vi "2DRasterScanWithScopeComm.vi"() -> ()   [LabVIEW 2015]
panel:
  out "error out 3":errorcluster
  out "error out 2":errorcluster
  in  "Z safe rretract":sgl
  in  "MG17Motor Z axis":refnum<k7>(container)
  in  "Home Z?":bool caption="Do this each time LabVIEW\n is opened, controllers are\n unplugged, or stages are\n         disconnected"
  in  "Z-Axis Serial":i32=27501169
  in  "Safe retract?":bool=TRUE
  in  "X safe rretract":sgl
  in  "Y safe retract":sgl
  out "Y error":errorcluster
  in  "Base filename":string="README" caption="Filename"
  in  "Save Each Point":bool=TRUE
  in  "X-Axis Serial":i32=45869591
  in  "Y-Axis Serial":i32=27501169
  out "Number of movements for Y stage":sgl=21.0
  in  "Distance from center X axis (mm)":dbl=15.0 step=0.001
  in  "Movement Step Size X axis (mm)":sgl=1.0 step=0.001
  in  "Channel Select":T1(ring)=enum."Channel 3"
  in  "Selected Directory":path=path "C:/Users/admin.WIN10DC20170225/Documents/Hydrophone Data/Test"
  in  "Stage Max Velocity (mm/s)":sgl=1.5
  in  "Stage Acceleration (mm/s²)":sgl=1.0
  in  "Stage Minimum Velocity (mm/s)":sgl
  in  "Center point Y axis (mm)":dbl=25.0 step=0.001 format="%#_13g"
  in  "Center point X axis (mm)":dbl=80.0 step=0.001 format="%#_13g"
  out "Number of movements for X stage":sgl=31.0
  in  "Distance from center Y axis (mm)":dbl=10.0 step=0.001
  in  "MG17Motor X axis":refnum<k7>(container)
  in  "Home stages\nbefore scanning":bool caption="Do this each time LabVIEW\n is opened, controllers are\n unplugged, or stages are\n         disconnected"
  in  "error in (no error)":errorcluster
  in  "MG17Motor Y axis":refnum<k7>(container)
  out "Current position in line":i32=1
  out "Current line number":i32=1
  in  "Movement Step Size Y axis (mm)":sgl=1.0 step=0.001
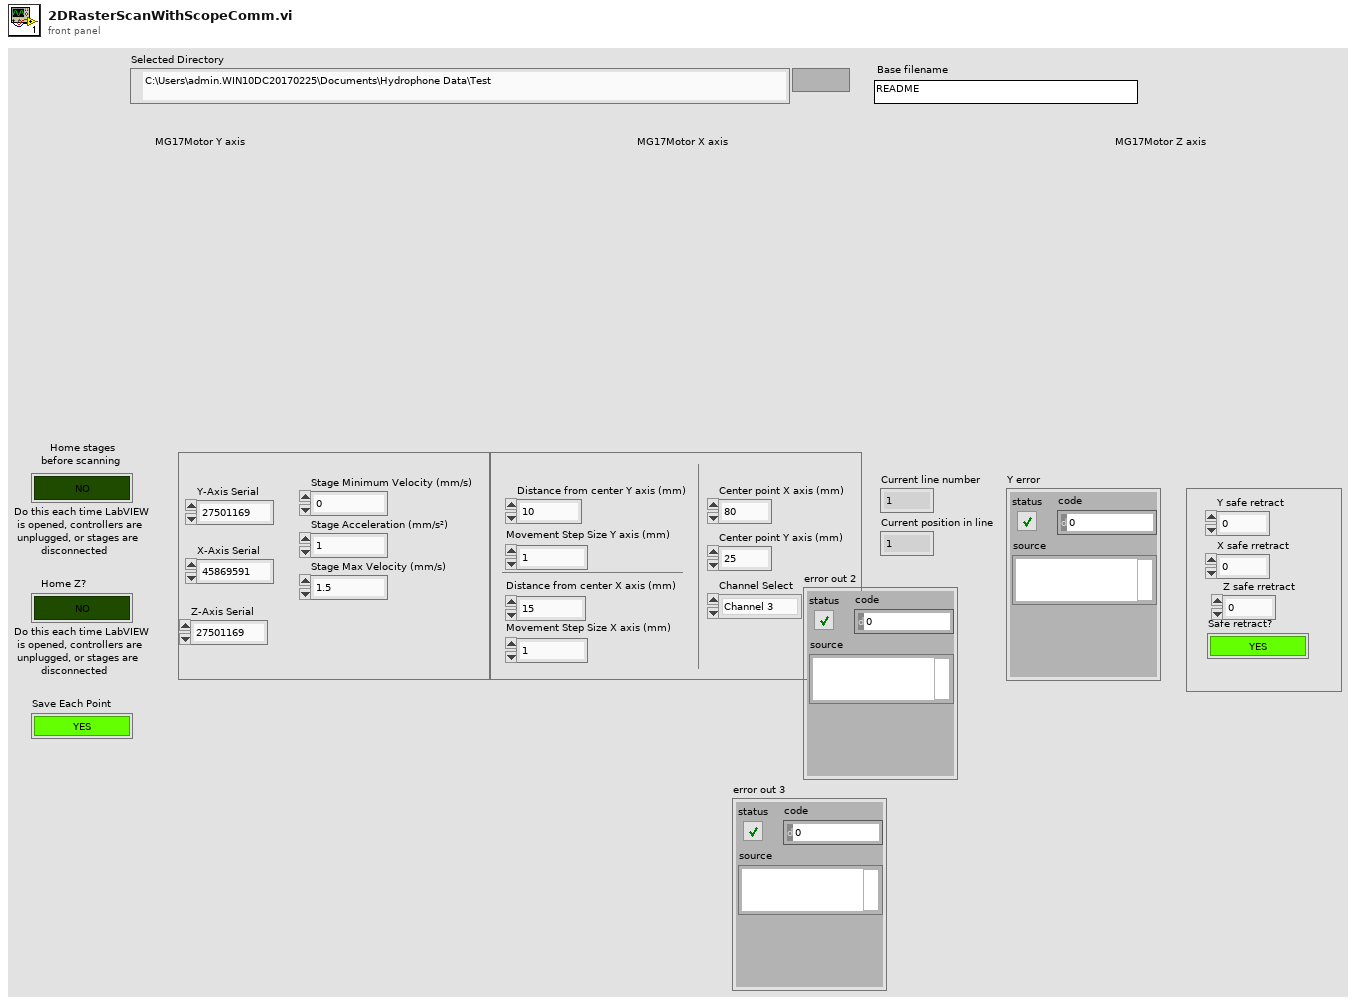
[diagram p1: front panel]
types:
  T1 = enum16{"Trace D", "Trace C", "Trace B", "Trace A", "Channel 4", "Channel 3", "Channel 2", "Channel 1"}
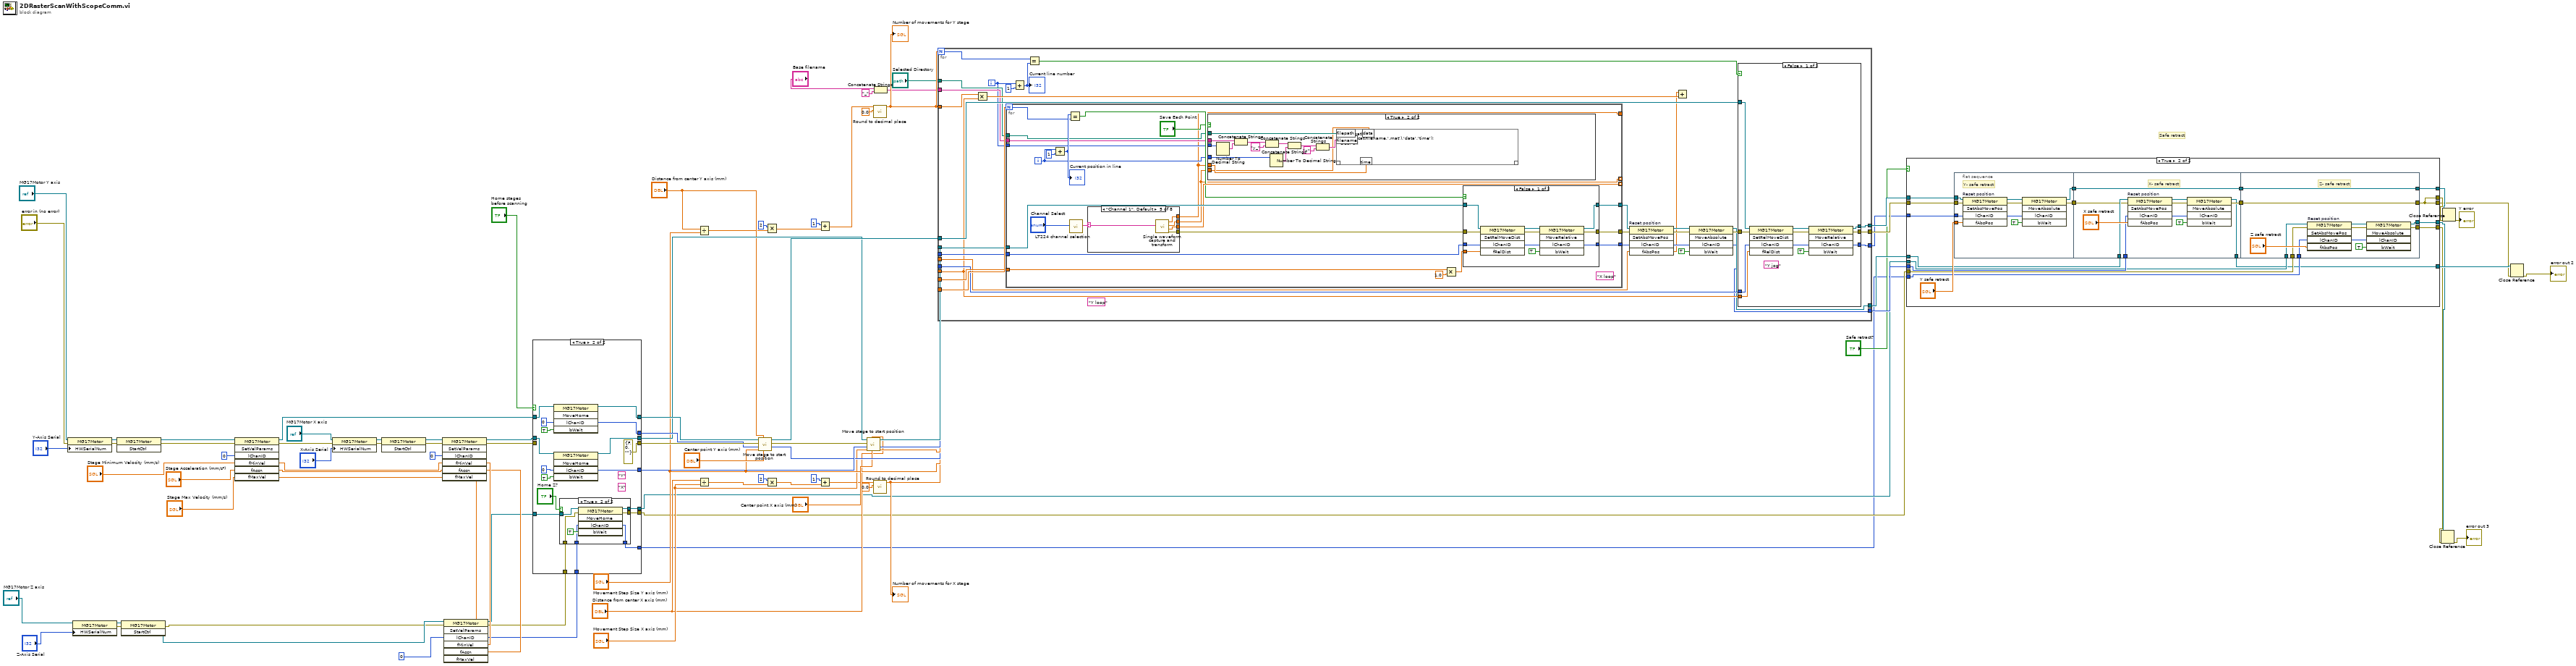
[diagram p0: block diagram]
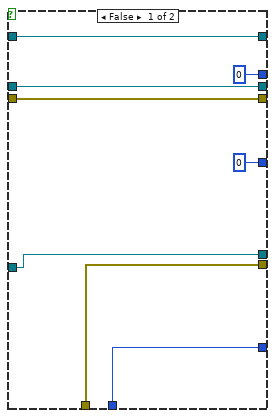
[diagram p3: hidden frame]
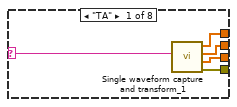
[diagram p8: hidden frame]
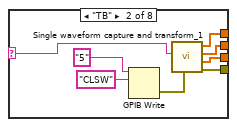
[diagram p9: hidden frame]
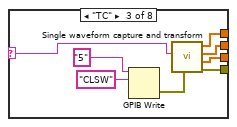
[diagram p10: hidden frame]
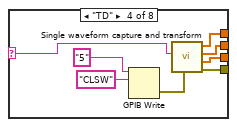
[diagram p11: hidden frame]
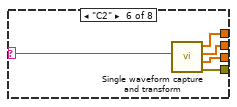
[diagram p12: hidden frame]
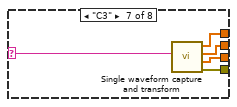
[diagram p13: hidden frame]
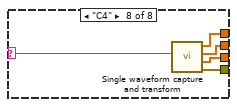
[diagram p14: hidden frame]
diagram:
  # "Safe retract"
  n1 = property on="Property Node" class="MG17Motor"(reference="MG17Motor Y axis", error in="error in (no error)", "HWSerialNum"="Y-Axis Serial") -> (reference out=w91:refnum<k7>, error out=w90:errorcluster)
  n2 = property on="Property Node" class="MG17Motor"(reference="MG17Motor Z axis", "HWSerialNum"="Z-Axis Serial") -> (reference out=w20:refnum<k7>, error out=w21:errorcluster)  [unwired: 1 in]
  n3 = invoke class="MG17Motor" method="StartCtrl"(reference=w91, error in=w90) -> (reference out=w83:refnum<k7>, error out=w84:errorcluster)  [unwired: 1 in, 1 out]
  n4 = invoke class="MG17Motor" method="StartCtrl"(reference=w20, error in=w21) -> (reference out=w15:refnum<k7>, error out=w14:errorcluster)  [unwired: 1 in, 1 out]
  n5 = invoke class="MG17Motor" method="SetVelParams"(reference=w83, error in=w84, "lChanID"=0, "fMinVel"="Stage Minimum Velocity (mm/s)", "fAccn"="Stage Acceleration (mm/s²)", "fMaxVel"="Stage Max Velocity (mm/s)") -> (reference out=w72:refnum<k7>, error out=w73:errorcluster, "fMinVel"=w53:sgl, "fAccn"=w52:sgl, "fMaxVel"=w51:sgl)  [unwired: 1 in, 2 out]
  n6 = property on="Property Node" class="MG17Motor"(reference="MG17Motor X axis", error in=w73, "HWSerialNum"="X-Axis Serial") -> (reference out=w86:refnum<k7>, error out=w85:errorcluster)
  n7 = invoke class="MG17Motor" method="StartCtrl"(reference=w86, error in=w85) -> (reference out=w82:refnum<k7>, error out=w75:errorcluster)  [unwired: 1 in, 1 out]
  n8 = invoke class="MG17Motor" method="SetVelParams"(reference=w82, error in=w75, "lChanID"=0, "fMinVel"=w53, "fAccn"=w52, "fMaxVel"=w51) -> (reference out=w81:refnum<k7>, error out=w74:errorcluster, "fMinVel"=w19:sgl, "fAccn"=w18:sgl, "fMaxVel"=w17:sgl)  [unwired: 1 in, 2 out]
  n9 = invoke class="MG17Motor" method="SetVelParams"(reference=w15, error in=w14, "lChanID"=0, "fMinVel"=w19, "fAccn"=w18, "fMaxVel"=w17) -> (reference out=w12:refnum<k7>, error out=w11:errorcluster, "lChanID"=w5:i32)  [unwired: 1 in, 4 out]
  n10 = case shown="True" "Home stages\nbefore scanning" {
    tunnel: [w97 w114] -> w62
    tunnel: [w98 w113] -> w68
    tunnel: [0 ("lChanID") w112] -> w63
    tunnel: [0 ("lChanID") w111] -> w66
    tunnel: [w96 errorcluster {"status"=FALSE, "code"=0, "source"=""} ("error out")] -> w67
    tunnel: w72 -> [w98 w109]
    tunnel: w81 -> [w97 w108]
    tunnel: w74 -> [w96 _]
    tunnel: w12 -> [w95 w106]
    tunnel: w11 -> [w94 w105]
    tunnel: [w95 w104] -> w9
    tunnel: [w94 w103] -> w8
    tunnel: w5 -> [w93 w102]
    tunnel: [w93 w101] -> w4
    frame False {
    }
    frame True {
      (unwired) "X"
      (unwired) "Y"
      n11 = invoke class="MG17Motor" method="MoveHome"(reference=w109, "lChanID"=0, "bWait"=TRUE) -> (reference out=w113:refnum<k7>, "lChanID"=w111:i32)  [unwired: 2 in, 3 out]
      n12 = invoke class="MG17Motor" method="MoveHome"(reference=w108, "lChanID"=0, "bWait"=TRUE) -> (reference out=w114:refnum<k7>, "lChanID"=w112:i32)  [unwired: 2 in, 3 out]
      n13 = case shown="True" "Home Z?" {
        tunnel: w106 -> [w121 w127]
        tunnel: w105 -> [w120 w126]
        tunnel: [w121 w125] -> w104
        tunnel: [w120 w124] -> w103
        tunnel: w102 -> [w119 w123]
        tunnel: [w119 w122] -> w101
        frame False {
        }
        frame True {
          n14 = invoke class="MG17Motor" method="MoveHome"(reference=w127, error in=w126, "lChanID"=w123, "bWait"=TRUE) -> (reference out=w125:refnum<k7>, error out=w124:errorcluster, "lChanID"=w122:i32)  [unwired: 1 in, 2 out]
        }
      }
    }
  }
  n15 = Divide(x="Distance from center Y axis (mm)", y="Movement Step Size Y axis (mm)") -> (x/y=w56:dbl)
  n16 = Divide(x="Distance from center X axis (mm)", y="Movement Step Size X axis (mm)") -> (x/y=w47:dbl)
  n17 = call "Move stage to start position.vi"("Center point of axis (mm)"="Center point Y axis (mm)", "Distance from center (mm)"="Distance from center Y axis (mm)", "Movement Step Size (mm)"="Movement Step Size Y axis (mm)", "lChanID"=w66, "error in"=w67, "reference in"=w68) -> ("lChanID out"=w57:i32, "error out"=w64:errorcluster, "reference out"=w65:refnum<k7>)  [unwired: 2 in, 1 out]
  n18 = Multiply(x=2, y=w56) -> (x*y=w70:dbl)
  n19 = Multiply(x=2, y=w47) -> (x*y=w48:dbl)
  n20 = Add(x=1, y=w70) -> (x+y=w40:dbl)
  n21 = Add(x=1, y=w48) -> (x+y=w41:dbl)
  n22 = call "Move stage to start position.vi"("Center point of axis (mm)"="Center point X axis (mm)", "Distance from center (mm)"="Distance from center X axis (mm)", "Movement Step Size (mm)"="Movement Step Size X axis (mm)", "lChanID"=w63, "error in"=w64, "reference in"=w62) -> ("Start position out"=w58:sgl, "lChanID out"=w59:i32, "reference out"=w60:refnum<k7>)  [unwired: 2 in, 1 out]
  n23 = call "Round to decimal place.vi"("Power of ten"=0.0, "Number to round"=w40) -> ("Rounded number"=w42:dbl)  [unwired: 8 in, 1 out]
  "Number of movements for Y stage" <- w42
  n24 = call "Round to decimal place.vi"("Power of ten"=0.0, "Number to round"=w41) -> ("Rounded number"=w43:dbl)  [unwired: 8 in, 1 out]
  "Number of movements for X stage" <- w43
  n25 = Concatenate Strings("Base filename", "_" ("string")) -> (w33:string)
  n26 = for {
    N: w42 -> [w149]
    tunnel: "Movement Step Size Y axis (mm)" -> [w154]
    tunnel: w43 -> [w159]
    tunnel: [w147] -> w30
    tunnel: [w146] -> w3
    tunnel: "Movement Step Size Y axis (mm)" -> [w139]
    tunnel: w65 -> [w145]
    tunnel: w60 -> [w144]
    tunnel: w59 -> [w143]
    tunnel: w58 -> [w142]
    tunnel: w57 -> [w141]
    tunnel: w42 -> [w138]
    tunnel: w33 -> [w134]
    tunnel: "Selected Directory" -> [w133]
    tunnel: [w131] -> w28
    tunnel: [w130] -> w29
    tunnel: [w129] -> w27
    i -> [w132]
    (unwired) "Y loop"
    n27 = Multiply(x=w138, y=w139) -> (x*y=w140:dbl)
    n28 = for {
      N: w159 -> [w181]
      tunnel: w154 -> [w188]
      tunnel: [w174] -> _
      tunnel: [w192] -> w135
      tunnel: [w193] -> w152
      tunnel: [w191] -> w151
      tunnel: [w185] -> _ mode=indexing
      tunnel: w144 -> [w189]
      tunnel: w143 -> [w190]
      tunnel: [w179] -> _ mode=indexing
      tunnel: w134 -> [w180]
      tunnel: w133 -> [w178]
      tunnel: w132 -> [w176]
      i -> [w177]
      (unwired) "X loop"
      n29 = Add(x=w177, y=1) -> (x+y=w182:i32)
      "Current position in line" <- w182
      n30 = Equal?(x=w182, y=w181) -> (x = y?=w183:bool)
      n31 = call "LT224 channel selection.vi"("Channel Select"="Channel Select") -> ("Selected channel"=w186:string)  [unwired: 10 in]
      n32 = case shown="\"Channel 1\", Default" w186 {
        selector: w186 -> [w226 w231 w239 w247 w255 w260 w265 w270]
        tunnel: [w229 w237 w245 w253 w258 w263 w268 w273] -> w184
        tunnel: [w228 w236 w244 w252 w257 w262 w267 w272] -> w185
        tunnel: [w227 w235 w243 w251 w256 w261 w266 w271] -> w174
        tunnel: [w225 w230 w238 w246 w254 w259 w264 w269] -> w179
        frame "TA" {
          n33 = call "Single waveform capture and transform_1.vi"("channel name (\"\")"=w226) -> ("error out"=w229:errorcluster, "Transformed waveform vector"=w228:dbl[], "waveform vector"=w225:dbl[], "Time vector"=w227:dbl[])  [unwired: 7 in]
        }
        frame "TB" {
          n34 = GPIB Write(0:"5" ("address string"), 1:"CLSW" ("data")) -> (6:w233:errorcluster)  [unwired: 3 in, 1 out]
          n35 = call "Single waveform capture and transform_1.vi"("error in"=w233, "channel name (\"\")"=w231) -> ("error out"=w237:errorcluster, "Transformed waveform vector"=w236:dbl[], "waveform vector"=w230:dbl[], "Time vector"=w235:dbl[])  [unwired: 6 in]
        }
        frame "TC" {
          n36 = GPIB Write(0:"5" ("address string"), 1:"CLSW" ("data")) -> (6:w241:errorcluster)  [unwired: 3 in, 1 out]
          n37 = call "Single waveform capture and transform.vi"("error in"=w241, "channel name (\"\")"=w239) -> ("error out"=w245:errorcluster, "Transformed waveform vector"=w244:dbl[], "waveform vector"=w238:dbl[], "Time vector"=w243:dbl[])  [unwired: 6 in]
        }
        frame "TD" {
          n38 = GPIB Write(0:"5" ("address string"), 1:"CLSW" ("data")) -> (6:w249:errorcluster)  [unwired: 3 in, 1 out]
          n39 = call "Single waveform capture and transform.vi"("error in"=w249, "channel name (\"\")"=w247) -> ("error out"=w253:errorcluster, "Transformed waveform vector"=w252:dbl[], "waveform vector"=w246:dbl[], "Time vector"=w251:dbl[])  [unwired: 6 in]
        }
        frame "Channel 1", Default {
          n40 = call "Single waveform capture and transform.vi"("channel name (\"\")"=w255) -> ("error out"=w258:errorcluster, "Transformed waveform vector"=w257:dbl[], "waveform vector"=w254:dbl[], "Time vector"=w256:dbl[])  [unwired: 7 in]
        }
        frame "C2" {
          n41 = call "Single waveform capture and transform.vi"("channel name (\"\")"=w260) -> ("error out"=w263:errorcluster, "Transformed waveform vector"=w262:dbl[], "waveform vector"=w259:dbl[], "Time vector"=w261:dbl[])  [unwired: 7 in]
        }
        frame "C3" {
          n42 = call "Single waveform capture and transform.vi"("channel name (\"\")"=w265) -> ("error out"=w268:errorcluster, "Transformed waveform vector"=w267:dbl[], "waveform vector"=w264:dbl[], "Time vector"=w266:dbl[])  [unwired: 7 in]
        }
        frame "C4" {
          n43 = call "Single waveform capture and transform.vi"("channel name (\"\")"=w270) -> ("error out"=w273:errorcluster, "Transformed waveform vector"=w272:dbl[], "waveform vector"=w269:dbl[], "Time vector"=w271:dbl[])  [unwired: 7 in]
        }
      }
      n44 = case shown="True" "Save Each Point" {
        tunnel: w180 -> [_ w202]
        tunnel: w179 -> [_ w197]
        tunnel: w178 -> [_ w200]
        tunnel: w177 -> [_ w210]
        tunnel: w176 -> [_ w204]
        tunnel: w174 -> [_ w198]
        frame False {
        }
        frame True {
          n45 = Number To Decimal String(number=w204) -> (decimal integer string=w201:string)  [unwired: 1 in]
          n46 = Concatenate Strings(w202, w201) -> (w209:string)
          n47 = Concatenate Strings(w209, "y_" ("string")) -> (w207:string)
          n48 = Number To Decimal String(number=w210) -> (decimal integer string=w203:string)  [unwired: 1 in]
          n49 = Concatenate Strings(w207, w203) -> (w205:string)
          n50 = Concatenate Strings(w205, "x" ("string")) -> (w199:string)
          n51 = script code="cd(filepath)\nsave(strcat(filename,'.mat'),'data','time');\nclear all"("filename"=w199, "filepath"=w200, "time"=w198, "data"=w197) -> ()  [unwired: 1 in, 1 out]
        }
      }
      n52 = Multiply(x=w188, y=sgl 1.0) -> (x*y=w195:sgl)
      n53 = case shown="False" w183 {
        tunnel: w195 -> [w221 _]
        tunnel: [w216 w222] -> w193
        tunnel: [w215 w224] -> w192
        tunnel: [w214 w223] -> w191
        tunnel: w190 -> [w213 w223]
        tunnel: w189 -> [w212 w222]
        tunnel: w184 -> [w211 w224]
        frame False {
          n54 = invoke class="MG17Motor" method="SetRelMoveDist"(reference=w212, error in=w211, "lChanID"=w213, "fRelDist"=w221) -> (reference out=w219:refnum<k7>, error out=w218:errorcluster, "lChanID"=w220:i32)  [unwired: 1 in, 2 out]
          n55 = invoke class="MG17Motor" method="MoveRelative"(reference=w219, error in=w218, "lChanID"=w220, "bWait"=TRUE) -> (reference out=w216:refnum<k7>, error out=w215:errorcluster, "lChanID"=w214:i32)  [unwired: 1 in, 2 out]
        }
        frame True {
        }
      }
    }
    n56 = Add(x=w132, y=1) -> (x+y=w136:i32)
    "Current line number" <- w136
    n57 = Equal?(x=w149, y=w136) -> (x = y?=w150:bool)
    n58 = invoke on="Reset position" class="MG17Motor" method="SetAbsMovePos"(reference=w152, error in=w135, "lChanID"=w151, "fAbsPos"=w142) -> (reference out=w155:refnum<k7>, error out=w157:errorcluster, "lChanID"=w156:i32, "fAbsPos"=w137:sgl)  [unwired: 1 in, 1 out]
    n59 = Add(x=w137, y=w140) -> ()  [unwired: 1 out]
    n60 = invoke class="MG17Motor" method="MoveAbsolute"(reference=w155, error in=w157, "lChanID"=w156, "bWait"=TRUE) -> (reference out=w130:refnum<k7>, error out=w148:errorcluster, "lChanID"=w129:i32)  [unwired: 1 in, 2 out]
    n61 = case shown="False" w150 {
      tunnel: w148 -> [w166 w173]
      tunnel: [w165 w171] -> w147
      tunnel: [w164 w173] -> w131
      tunnel: [w163 w172] -> w146
      tunnel: w139 -> [w162 _]
      tunnel: w145 -> [w161 w171]
      tunnel: w141 -> [w160 w172]
      frame False {
        (unwired) "Y jog"
        n62 = invoke class="MG17Motor" method="SetRelMoveDist"(reference=w161, error in=w166, "lChanID"=w160, "fRelDist"=w162) -> (reference out=w168:refnum<k7>, error out=w169:errorcluster, "lChanID"=w167:i32)  [unwired: 1 in, 2 out]
        n63 = invoke class="MG17Motor" method="MoveRelative"(reference=w168, error in=w169, "lChanID"=w167, "bWait"=TRUE) -> (reference out=w165:refnum<k7>, error out=w164:errorcluster, "lChanID"=w163:i32)  [unwired: 1 in, 2 out]
      }
      frame True {
      }
    }
  }
  n64 = case shown="True" "Safe retract?" {
    tunnel: w30 -> [w278 w296]
    tunnel: w29 -> [w277 w290]
    tunnel: w28 -> [w276 w294]
    tunnel: w27 -> [_ w288]
    tunnel: [w278 w293] -> w26
    tunnel: [w276 w279] -> w25
    tunnel: [w277 w280] -> w24
    tunnel: [w276 w279] -> w23
    tunnel: w9 -> [w275 w284]
    tunnel: w8 -> [w274 w283]
    tunnel: [w275 w285] -> w7
    tunnel: [w274 w281] -> w6
    tunnel: w4 -> [_ w282]
    tunnel: w3 -> [_ w289]
    frame False {
    }
    frame True {
      n65 = flat-sequence {
        tunnel: w296 -> [w302]
        tunnel: "Y safe retract" -> [w301]
        tunnel: w294 -> [w300]
        tunnel: [w299] -> w292
        tunnel: [w298] -> w291
        tunnel: w289 -> [w297]
        tunnel: w292 -> [w310]
        tunnel: w291 -> [w309]
        tunnel: w290 -> [w312]
        tunnel: w288 -> [w311]
        tunnel: [w310] -> w287
        tunnel: [w308] -> w286
        tunnel: [w307] -> w280
        tunnel: [w318] -> w279
        tunnel: [w329] -> w293
        tunnel: w287 -> [w329]
        tunnel: w286 -> [w318]
        tunnel: [w323] -> w285
        tunnel: w284 -> [w322]
        tunnel: w283 -> [w321]
        tunnel: w282 -> [w320]
        tunnel: [w319] -> w281
        frame #0 {
          # "Y- safe retract"
          n66 = invoke on="Reset position" class="MG17Motor" method="SetAbsMovePos"(reference=w302, error in=w300, "lChanID"=w297, "fAbsPos"=w301) -> (reference out=w306:refnum<k7>, error out=w305:errorcluster, "lChanID"=w304:i32)  [unwired: 1 in, 2 out]
          n67 = invoke class="MG17Motor" method="MoveAbsolute"(reference=w306, error in=w305, "lChanID"=w304, "bWait"=TRUE) -> (reference out=w299:refnum<k7>, error out=w298:errorcluster)  [unwired: 1 in, 3 out]
        }
        frame #1 {
          # "X- safe retract"
          n68 = invoke on="Reset position" class="MG17Motor" method="SetAbsMovePos"(reference=w312, error in=w309, "lChanID"=w311, "fAbsPos"="X safe rretract") -> (reference out=w313:refnum<k7>, error out=w314:errorcluster, "lChanID"=w317:i32)  [unwired: 1 in, 2 out]
          n69 = invoke class="MG17Motor" method="MoveAbsolute"(reference=w313, error in=w314, "lChanID"=w317, "bWait"=TRUE) -> (reference out=w307:refnum<k7>, error out=w308:errorcluster)  [unwired: 1 in, 3 out]
        }
        frame #2 {
          # "Z- safe retract"
          n70 = invoke on="Reset position" class="MG17Motor" method="SetAbsMovePos"(reference=w322, error in=w321, "lChanID"=w320, "fAbsPos"="Z safe rretract") -> (reference out=w324:refnum<k7>, error out=w325:errorcluster, "lChanID"=w326:i32)  [unwired: 1 in, 2 out]
          n71 = invoke class="MG17Motor" method="MoveAbsolute"(reference=w324, error in=w325, "lChanID"=w326, "bWait"=TRUE) -> (reference out=w323:refnum<k7>, error out=w319:errorcluster)  [unwired: 1 in, 3 out]
        }
      }
    }
  }
  n72 = Close Reference(reference=w7, error in (no error)=w6) -> (error out=→"error out 3":errorcluster)
  n73 = Close Reference(reference=w26, error in (no error)=w25) -> (error out=→"Y error":errorcluster)
  n74 = Close Reference(reference=w24, error in (no error)=w23) -> (error out=→"error out 2":errorcluster)
